vi "Sorter (Initial, without Timer).vi"() -> ()   [LabVIEW 2014]
panel:
  in  "D0":bool
  in  "D1":bool
  in  "Start/Stop":bool
  out "M0-":bool
  out "M0+":bool
  out "W1":bool
  out "W4":bool
  out "W0":bool
  out "M1-":bool
  out "M1+":bool
  out "M4-":bool
  out "M4+":bool
  # "Sorter Control Panel"
  # "Belt 1"
  # "#11"
  # "#10"
  # "Belt 0"
  # "Belt 4"
  # "#00"
  # "#01"
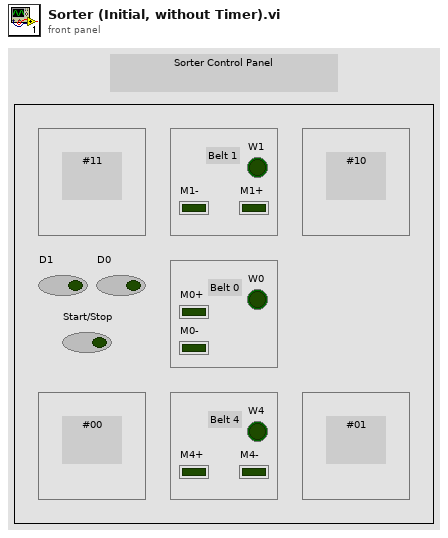
[diagram p1: front panel]
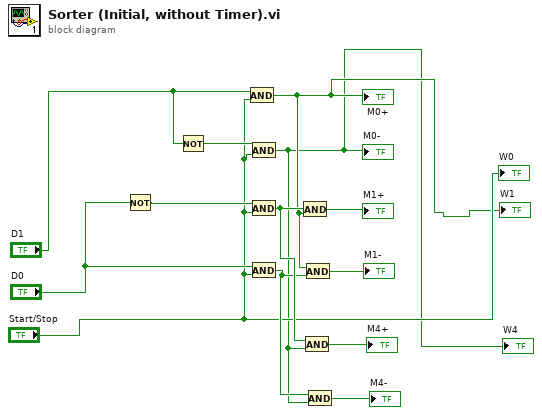
[diagram p0: block diagram]
diagram:
  n1 = Not(x="D0") -> (.not. x?=w11:bool)
  n2 = Not(x="D1") -> (.not. x?=w13:bool)
  n3 = And(x="D1", y="Start/Stop") -> (x .and. y?=w2:bool)
  "W1" <- w2
  "M0+" <- w2
  n4 = And(x=w13, y="Start/Stop") -> (x .and. y?=w1:bool)
  "W4" <- w1
  "M0-" <- w1
  n5 = And(x=w11, y="Start/Stop") -> (x .and. y?=w6:bool)
  n6 = And(x="D0", y="Start/Stop") -> (x .and. y?=w4:bool)
  n7 = And(x=w6, y=w2) -> (x .and. y?=→"M1+":bool)
  n8 = And(x=w6, y=w1) -> (x .and. y?=→"M4+":bool)
  n9 = And(x=w2, y=w4) -> (x .and. y?=→"M1-":bool)
  n10 = And(x=w4, y=w1) -> (x .and. y?=→"M4-":bool)
  "W0" <- "Start/Stop"
